vi "dice.vi"() -> ()   [LabVIEW 2019]
panel:
  out "Pict Ring":u16(ring)
  out "Array":string[](array[string])
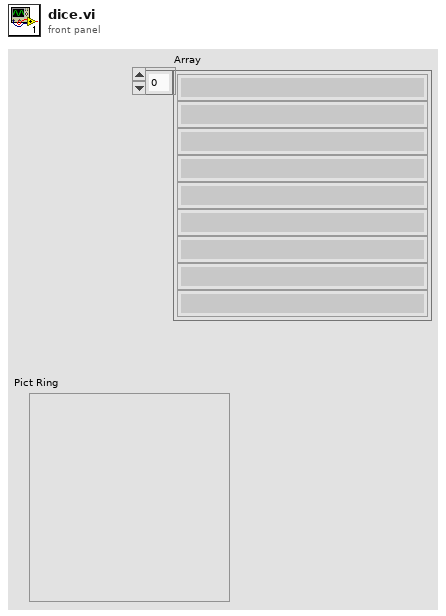
[diagram p1: front panel]
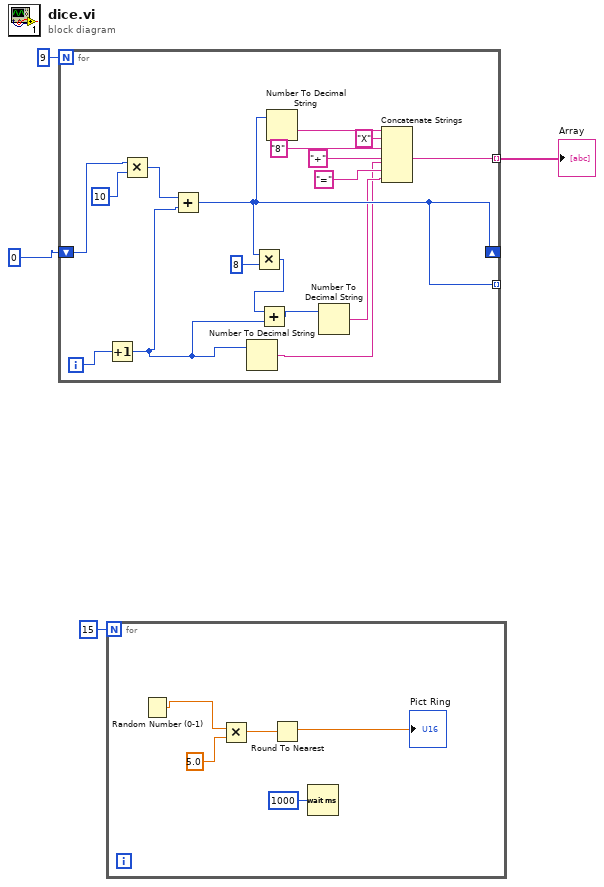
[diagram p0: block diagram]
diagram:
  n1 = for {
    N: 9 -> [_]
    shift-right: [w13] -> _
    shift-left: 0 -> [w21]
    tunnel: [w13] -> _ mode=indexing
    tunnel: [w7] -> w2 mode=indexing
    i -> [w19]
    n2 = Increment(x=w19) -> (x+1=w14:i32)
    n3 = Multiply(x=w21, y=10) -> (x*y=w18:i32)
    n4 = Add(x=w18, y=w14) -> (x+y=w13:i32)
    n5 = Number To Decimal String(number=w14) -> (decimal integer string=w5:string)  [unwired: 1 in]
    n6 = Multiply(x=w13, y=8) -> (x*y=w16:i32)
    n7 = Add(x=w16, y=w14) -> (x+y=w15:i32)
    n8 = Number To Decimal String(number=w13) -> (decimal integer string=w12:string)  [unwired: 1 in]
    n9 = Number To Decimal String(number=w15) -> (decimal integer string=w6:string)  [unwired: 1 in]
    n10 = Concatenate Strings(w12, "X" ("string"), "8" ("string"), "+" ("string"), w5, "=" ("string"), w6) -> (w7:string)
  }
  "Array" <- w2
  n11 = for {
    N: 15 -> [_]
    n12 = Random Number (0-1)() -> (number: 0 to 1=w26:dbl)
    n13 = Multiply(x=w26, y=5.0) -> (x*y=w24:dbl)
    n14 = Round To Nearest(number=w24) -> (nearest integer value=→"Pict Ring":dbl)
    n15 = Wait (ms)(milliseconds to wait=u32 1000) -> ()  [unwired: 1 out]
  }
